vi "3.2 Real Units for Motors.vi"(0 "Numeric":i32, 1 "Numeric 2":i32, 2 "2.1 Act Debug.Lidar.Lidar Position Integer":i32, 3 "2.1 Act Debug.Steering.Steering Position Integer":i32, 6 "2.1 Act Debug.Drive.Drive Position Integer":i32) -> (4 "Lidar Velocity":dbl, 5 "Lidar Position":dbl, 7 "Steering Velocity":dbl, 8 "Steering Position":dbl, 9 "Drive Velocity":dbl, 10 "Drive Position":dbl)   [LabVIEW 2010]
uses:
  3.0-Global.vi
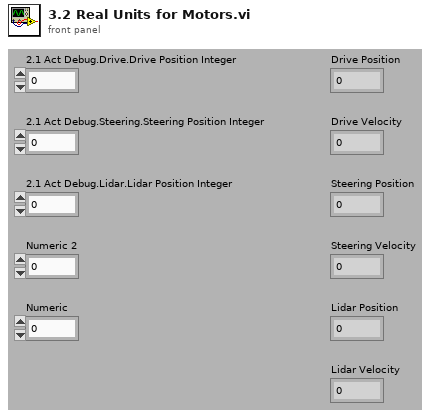
[diagram p1: front panel]
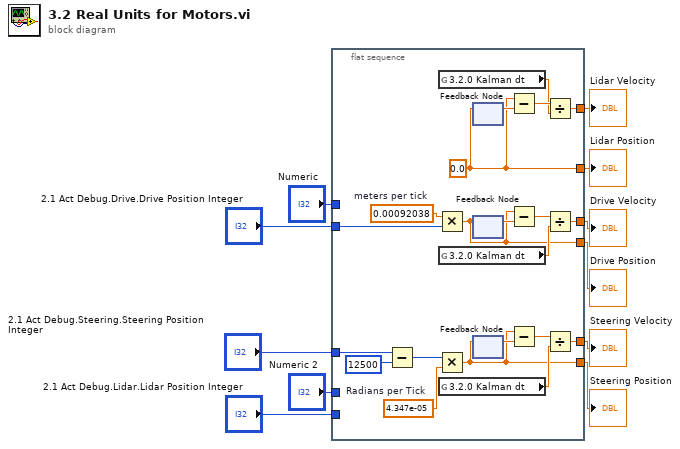
[diagram p0: block diagram]
diagram:
  n1 = flat-sequence {
    tunnel: "2.1 Act Debug.Drive.Drive Position Integer" -> [w18]
    tunnel: "2.1 Act Debug.Steering.Steering Position Integer" -> [w16]
    tunnel: "2.1 Act Debug.Lidar.Lidar Position Integer" -> [_]
    tunnel: [w17] -> w5
    tunnel: [w20] -> w6
    tunnel: [w12] -> w7
    tunnel: [w22] -> w8
    tunnel: [w21] -> w9
    tunnel: "Numeric 2" -> [_]
    tunnel: "Numeric" -> [_]
    tunnel: [w30] -> w1
    frame #0 {
      w13 = 4.347e-05  # Radians per Tick
      w19 = 0.00092038  # meters per tick
      w22 = 0.0
      n2 = Subtract(x=w16, y=12500) -> (x-y=w14:i32)
      n3 = Multiply(x=w19, y=w18) -> (x*y=w17:dbl)
      n4 = Multiply(x=w14, y=w13) -> (x*y=w12:dbl)
      n5 = global read "3.0-Global.vi" "3.2.0 Kalman dt"() -> (w23:dbl)
      n6 = global read "3.0-Global.vi" "3.2.0 Kalman dt"() -> (w28:dbl)
      n7 = global read "3.0-Global.vi" "3.2.0 Kalman dt"() -> (w29:dbl)
      n8 = feedback #1() -> (w25:dbl)  [unwired: 1 in]
      n9 = feedback-in #1(w22) -> ()
      n10 = feedback #2() -> (w26:dbl)  [unwired: 1 in]
      n11 = feedback-in #2(w17) -> ()
      n12 = feedback-in #3(w12) -> ()
      n13 = feedback #3() -> (w32:dbl)  [unwired: 1 in]
      n14 = Subtract(x=w22, y=w25) -> (x-y=w24:dbl)
      n15 = Subtract(x=w17, y=w26) -> (x-y=w27:dbl)
      n16 = Subtract(x=w12, y=w32) -> (x-y=w31:dbl)
      n17 = Divide(x=w24, y=w23) -> (x/y=w21:dbl)
      n18 = Divide(x=w27, y=w28) -> (x/y=w20:dbl)
      n19 = Divide(x=w31, y=w29) -> (x/y=w30:dbl)
    }
  }
  "Lidar Velocity" <- w9
  "Lidar Position" <- w8
  "Steering Velocity" <- w1
  "Steering Position" <- w7
  "Drive Velocity" <- w6
  "Drive Position" <- w5
